vi "ExecStepCmd.vi"(9 "SP_CHAMBER":dbl, 10 "SP_DUT":dbl, 11 "Stand in":refnum<class "Stand.lvclass">) -> (3 "Stand out":refnum<class "Stand.lvclass">)   [LabVIEW 2019, in "Stand.lvclass"]
uses:
  Stand.lvclass
  Stand.lvclass/Stand.ctl
  TypeDef/Direction.ctl
  TypeDef/Mode.ctl
  TypeDef/ExecuteStepState.ctl
  AI_class/AI.lvclass
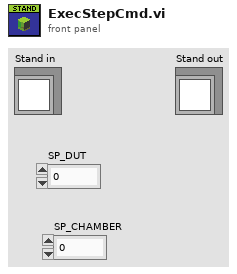
[diagram p1: front panel]
types:
  T1 = typedef "Direction.ctl" = enum8{"DUT", "Chamber"}
  T2 = typedef "AI_Data.ctl" = cluster{"Stat Data":T3, "OutOfRangeMax":bool, "OutOfRangeMin":bool, "HIHI":bool, "HI":bool, "LO":bool, "LOLO":bool}
  T3 = typedef "AI Statistics Data.ctl" = cluster{"raw mean":dbl, "scl mean":dbl, "raw mean 1Hz":dbl, "scl mean 1Hz":dbl}
  T4 = typedef "SP_TYPE.ctl" = enum16{"ERROR", "ZIRO", "BASE", "SP"}
  T5 = typedef "ExecuteStepState.ctl" = enum16{"Init", "Set: Backpressure ", "Preload: HI", "Set: HI", "Maintenance: HI", "Down: Pressure", "BLOCK"}
  T6 = typedef "Mode.ctl" = enum16{"IDLE", "FILLING", "EXECUTE_SP", "DRAIN"}
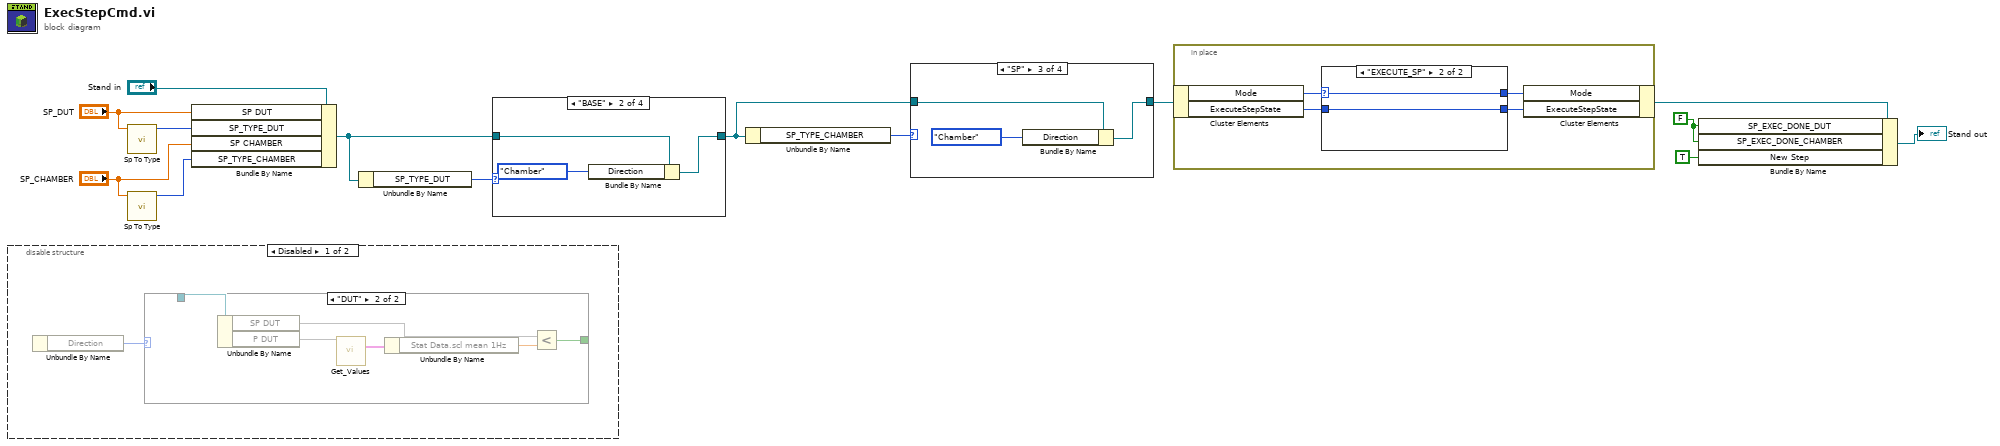
[diagram p0: block diagram]
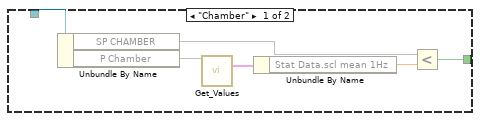
[diagram p2: hidden frame]
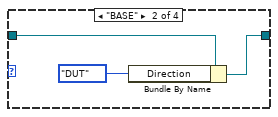
[diagram p5: hidden frame]
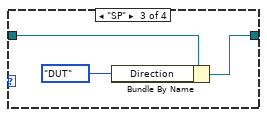
[diagram p8: hidden frame]
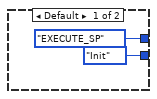
[diagram p10: hidden frame]
diagram:
  w3 = FALSE ("Data.STS.SP_EXEC_DONE_DUT")
  n1 = disable-structure shown="Disabled" {
    frame Disabled {
      n2 = Unbundle By Name() -> ("Direction"=w15:T1)  [unwired: 1 in]
      n3 = case shown="\"DUT\"" w15 {
        tunnel: [w18 w24] -> _
        tunnel: _ -> [w17 w23]
        frame "Chamber" {
          n4 = Unbundle By Name(w17) -> ("SP CHAMBER"=w16, "P Chamber"=w20)
          n5 = call "Get_Values.vi"("reference in"=w20) -> ("Data"=w21:T2)  [unwired: 14 in]
          n6 = Unbundle By Name(w21) -> ("Stat Data.scl mean 1Hz"=w19:dbl)
          n7 = Less?(x=w16, y=w19) -> (x < y?=w18:bool)
        }
        frame "DUT" {
          n8 = Unbundle By Name(w23) -> ("SP DUT"=w22, "P DUT"=w26)
          n9 = call "Get_Values.vi"("reference in"=w26) -> ("Data"=w27:T2)  [unwired: 14 in]
          n10 = Unbundle By Name(w27) -> ("Stat Data.scl mean 1Hz"=w25:dbl)
          n11 = Less?(x=w22, y=w25) -> (x < y?=w24:bool)
        }
      }
    }
    frame Enabled {
    }
  }
  n12 = call "Sp To Type.vi"("SP DUT"="SP_DUT") -> ("Sp_type"=w13:T4)  [unwired: 14 in]
  n13 = call "Sp To Type.vi"("SP DUT"="SP_CHAMBER") -> ("Sp_type"=w11:T4)  [unwired: 14 in]
  n14 = Bundle By Name(cluster="Stand in", "SP DUT"="SP_DUT", "SP_TYPE_DUT"=w13, "SP CHAMBER"="SP_CHAMBER", "SP_TYPE_CHAMBER"=w11) -> (w5:refnum<class "Stand.lvclass">)
  n15 = Unbundle By Name(w5) -> ("SP_TYPE_DUT"=w10:T4)
  n16 = case shown="\"BASE\"" w10 {
    tunnel: w5 -> [w28 w31 w34 w35]
    tunnel: [w28 w30 w33 w35] -> w7
    frame "ERROR" {
    }
    frame "BASE" {
      n17 = Bundle By Name(cluster=w31, "Direction"=Direction."Chamber" ("Data.Direction")) -> (w30:refnum<class "Stand.lvclass">)
    }
    frame "SP" {
      n18 = Bundle By Name(cluster=w34, "Direction"=Direction."DUT" ("Data.Direction")) -> (w33:refnum<class "Stand.lvclass">)
    }
    frame "ZIRO" {
    }
  }
  n19 = Unbundle By Name(w7) -> ("SP_TYPE_CHAMBER"=w8:T4)
  n20 = case shown="\"SP\"" w8 {
    tunnel: w7 -> [w36 w39 w42 w43]
    tunnel: [w36 w38 w41 w43] -> w6
    frame "ERROR" {
    }
    frame "BASE" {
      n21 = Bundle By Name(cluster=w39, "Direction"=Direction."DUT" ("Data.Direction")) -> (w38:refnum<class "Stand.lvclass">)
    }
    frame "SP" {
      n22 = Bundle By Name(cluster=w42, "Direction"=Direction."Chamber" ("Data.Direction")) -> (w41:refnum<class "Stand.lvclass">)
    }
    frame "ZIRO" {
    }
  }
  n23 = in-place {
    n24 = in-place-cluster #1(w6) -> ("Mode"=w47:T6, "ExecuteStepState"=w44:T5)
    n25 = case shown="\"EXECUTE_SP\"" w47 {
      selector: w47 -> [_ w51]
      tunnel: [Mode."EXECUTE_SP" ("Mode") w51] -> w46
      tunnel: [ExecuteStepState."Init" ("Data.ExecuteStepState") w50] -> w45
      tunnel: w44 -> [_ w50]
      frame Default {
      }
      frame "EXECUTE_SP" {
      }
    }
    n26 = in-place-cluster #1("Mode"=w46, "ExecuteStepState"=w45) -> (w4:refnum<class "Stand.lvclass">)
  }
  n27 = Bundle By Name(cluster=w4, "SP_EXEC_DONE_DUT"=w3, "SP_EXEC_DONE_CHAMBER"=w3, "New Step"=TRUE ("Data.New Step")) -> (→"Stand out":refnum<class "Stand.lvclass">)
